vi "Class - ResultCntr.AddResultID.vi"(8 "error in (no error)":errorcluster, 11 "Class - ResultCntr in":refnum<class "Class - ResultCntr.lvclass">) -> (0 "error out":errorcluster, 1 "ID":string, 3 "Class - ResultCntr out":refnum<class "Class - ResultCntr.lvclass">)   [LabVIEW 2024, in "EQMF.lvlib" / "Results.lvlib" / "Class - ResultCntr.lvclass"]
uses:
  Class - ResultCntr.lvclass
  Class - ResultCntr.lvclass/Class - ResultCntr.ctl
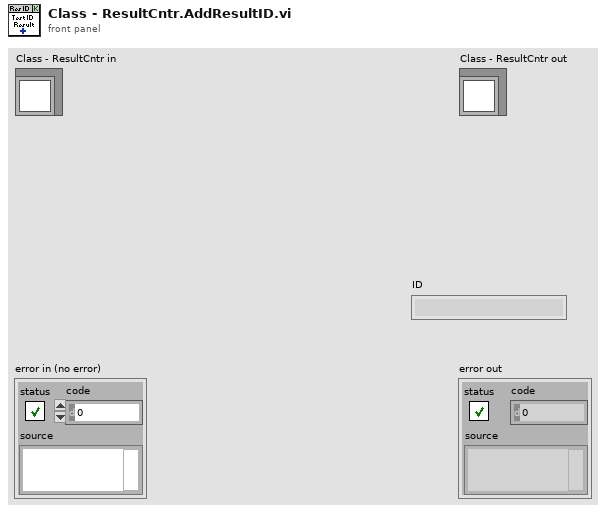
[diagram p1: front panel]
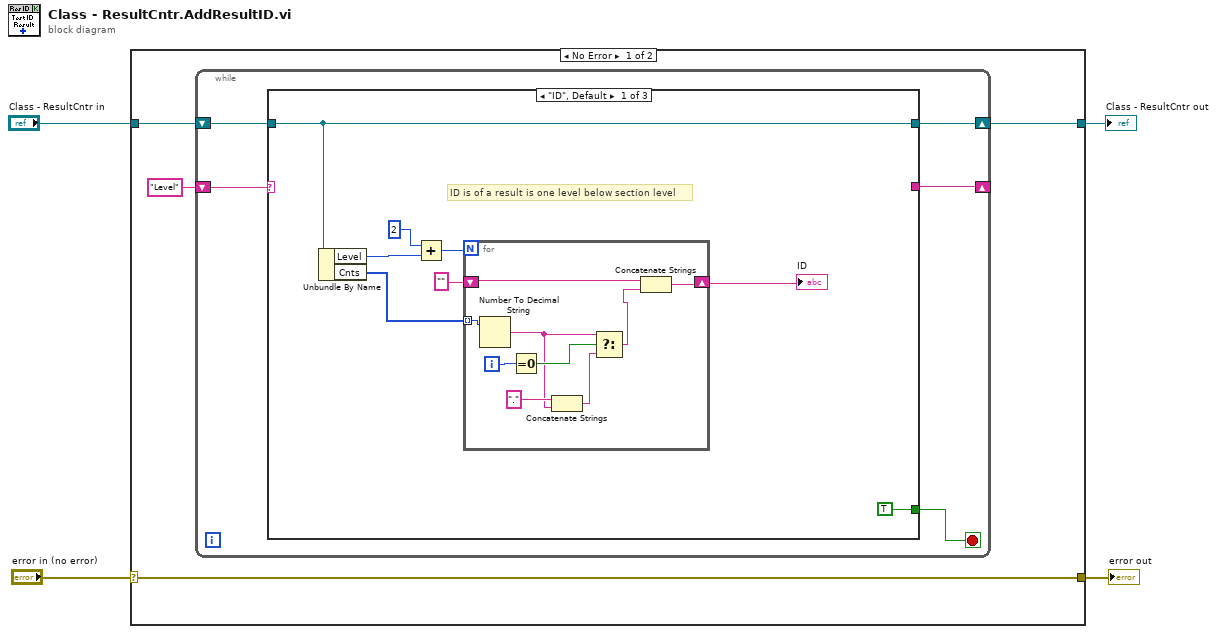
[diagram p0: block diagram]
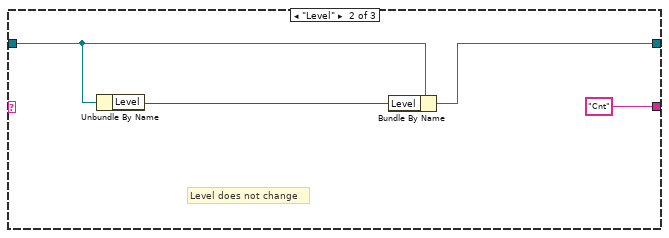
[diagram p2: hidden frame]
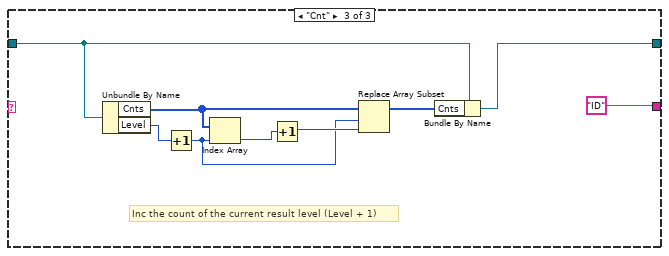
[diagram p3: hidden frame]
diagram:
  n1 = case shown="No Error" "error in (no error)" {
    selector: "error in (no error)" -> [w8 w45]
    tunnel: [w8 w45] -> w3
    tunnel: [w5 w44] -> w1
    tunnel: "Class - ResultCntr in" -> [w7 w44]
    frame No Error {
      n2 = while {
        shift-right: [w11] -> w5
        shift-left: w7 -> [w12]
        shift-right: [w10] -> _
        shift-left: "Level" -> [w13]
        stop <- w9 stop-if-true
        n3 = case shown="\"ID\", Default" w13 {
          tunnel: w12 -> [w19 w33 w42]
          tunnel: [w19 w32 w41] -> w11
          tunnel: [_ "Cnt" "ID"] -> w10
          tunnel: [TRUE _ _] -> w9
          frame "ID", Default {
            # "ID is of a result is one level below section level"
            n4 = Unbundle By Name(w19) -> ("Level"=w15:i32, "Cnts"=w18:i32[])
            n5 = Add(x=2, y=w15) -> (x+y=w16:i32)
            n6 = for {
              N: w16 -> [_]
              tunnel: w18 -> [w29] mode=indexing
              shift-right: [w24] -> w17
              shift-left: "" -> [w23]
              i -> [w30]
              n7 = Number To Decimal String(number=w29) -> (decimal integer string=w25:string)  [unwired: 1 in]
              n8 = Equal To 0?(x=w30) -> (x = 0?=w26:bool)
              n9 = Concatenate Strings(".", w25) -> (w27:string)
              n10 = Select(t=w25, s=w26, f=w27) -> (s? t:f=w22:string)
              n11 = Concatenate Strings(w23, w22) -> (w24:string)
            }
            "ID" <- w17
          }
          frame "Level" {
            # "Level does not change"
            n12 = Unbundle By Name(w33) -> ("Level"=w31:i32)
            n13 = Bundle By Name(cluster=w33, "Level"=w31) -> (w32:refnum<class "Class - ResultCntr.lvclass">)
          }
          frame "Cnt" {
            # "Inc the count of the current result level (Level + 1)"
            n14 = Unbundle By Name(w42) -> ("Cnts"=w38:i32[], "Level"=w36:i32)
            n15 = Increment(x=w36) -> (x+1=w35:i32)
            n16 = Index Array(array=w38, index=w35) -> (element=w37:i32)
            n17 = Increment(x=w37) -> (x+1=w39:i32)
            n18 = Replace Array Subset(array=w38, new element=w39, index=w35) -> (w40:i32[])
            n19 = Bundle By Name(cluster=w42, "Cnts"=w40) -> (w41:refnum<class "Class - ResultCntr.lvclass">)
          }
        }
      }
    }
    frame Error {
    }
  }
  "error out" <- w3
  "Class - ResultCntr out" <- w1
